vi "SSR_Create.vi"(0 "reference in":refnum<class "SSR.lvclass">, 5 "error in (no error)":errorcluster) -> (14 "reference out":refnum<class "SSR.lvclass">, 19 "error out":errorcluster)   [LabVIEW 2017, in "SSR.lvclass"]
uses:
  SSR.lvclass
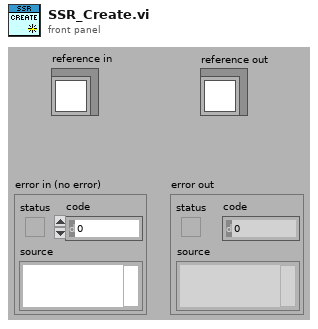
[diagram p1: front panel]
types:
  T1 = typedef "SSR.lvclass/ObjectAttributes.ctl" = cluster{"SSR Task":refnum<k21>, "SSR On/Off Status":bool, "Number of SSR Modules":u32, "Number of Total SSR Channels":u32, "SSR Module Names (NI-Max Name)":string[], "Number of Channels Per SSR Module":i32[], "SSR Status":bool[], "SSR Status to Set":bool[], "SSR VI Reference":refnum<vi>}
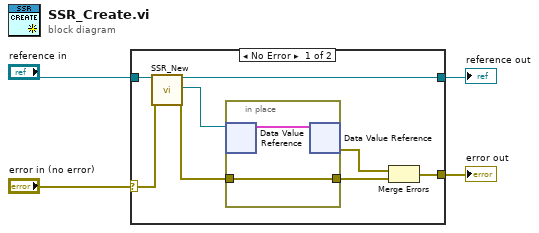
[diagram p0: block diagram]
diagram:
  n1 = case shown="No Error" "error in (no error)" {
    selector: "error in (no error)" -> [w11 w16]
    tunnel: [w8 w16] -> w3
    tunnel: "reference in" -> [w12 w15]
    tunnel: [w10 w15] -> w1
    frame No Error {
      n2 = call "SSR_New.vi"("reference in"=w12, "error in (no error)"=w11) -> ("reference out"=w10:refnum<class "SSR.lvclass">, "DVRRefOut"=w7:refnum<data-value>, "error out"=w6:errorcluster)  [unwired: 14 in, 1 out]
      n3 = in-place {
        in-place-border: w6 -> [w14]
        in-place-border: [w14] -> w5
        n4 = in-place-dvr #1(w7) -> (w13:T1)  [unwired: 1 out]
        n5 = in-place-dvr #1(w13) -> (w9:errorcluster)  [unwired: 1 out]
      }
      n6 = Merge Errors(w9, w5) -> (w8:errorcluster)
    }
    frame Error {
    }
  }
  "error out" <- w3
  "reference out" <- w1
